vi "test-FlyWheel-Sim-Test2.vi"() -> (3 "All Passed":bool)   [LabVIEW 2019]
uses:
  <vilib>/Analysis/Matrix/Datatypes/RealMatrix.ctl
  <vilib>/Analysis/Matrix/NI_Matrix.lvlib
  <vilib>/Rock Robotics/WPI/ThirdParty/JAS_Junk/TrajLib/Trajectory_Library.lvlib
  <vilib>/Rock Robotics/WPI/ThirdParty/JAS_Junk/TrajLib/DCMotor_GetCIM.vi
panel:
  out "Speed Control Passed":bool
  out "Speed Ctrl":T1(graph)
  out "Error":bool
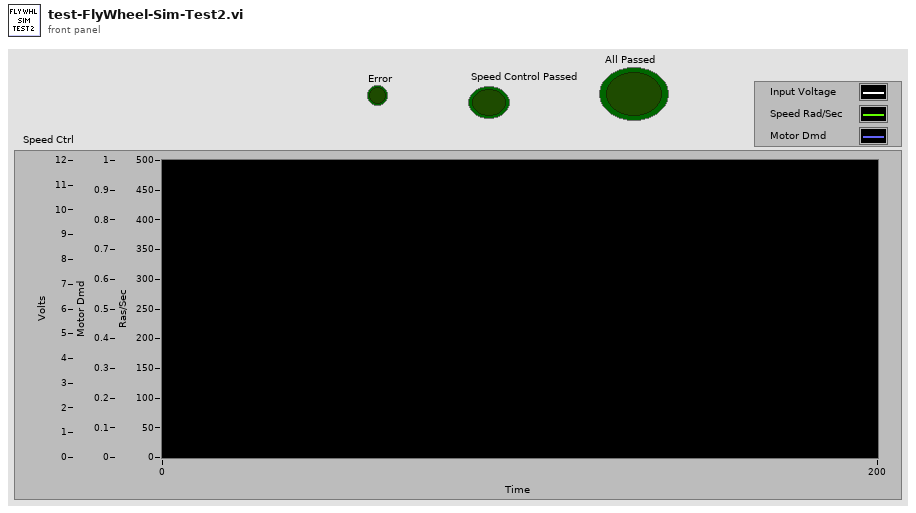
[diagram p1: front panel]
types:
  T1 = cluster{dbl, "Velocity_RadPerSec":dbl, "upper limit":dbl}
  T2 = typedef "NI_Matrix.lvlib/RealMatrix.ctl" = dbl[][]
  T3 = typedef "Trajectory_Library.lvlib/DCMOTOR.CTL" = cluster{"nominalVoltage_Volts":dbl, "StallTorque_NM":dbl, "StallCurrent_Amps":dbl, "FreeCurrent_Amps":dbl, "FreeSpeed_RadPerSec":dbl, "R_Ohms":dbl, "KvINV_RadPerSecPerVolt":dbl, "Kt_NMPerAmp":dbl, "L_H":dbl, "Jr_KgM2":dbl}
  T4 = typedef "Trajectory_Library.lvlib/FLYWHEEL_SIM.ctl" = cluster{"LinearSystemSim":T5, "GearBox":T3, "Gearing":dbl}
  T5 = typedef "Trajectory_Library.lvlib/LINEAR_SYSTEM_SIM.ctl" = cluster{"m_Plant":T6, "m_X":T2, "m_Y":T2, "m_U":T2, "MeasureStdDev":T2}
  T6 = typedef "Trajectory_Library.lvlib/LINEAR_SYSTEM.ctl" = cluster{"m_A":T2, "m_B":T2, "m_C":T2, "m_D":T2, "States":i32, "Inputs":i32, "Outputs":i32}
  T7 = typedef "Trajectory_Library.lvlib/PID_TUNING.ctl" = cluster{"Kp":dbl, "Ki":dbl, "Kd":dbl, "MaximumIntegral":dbl, "MinimumIntegral":dbl, "IntegralZone":dbl}
  T8 = typedef "Trajectory_Library.lvlib/PID_INPUT_LIMITS.ctl" = cluster{"MaxInput":dbl, "MinInput":dbl, "Continuous":bool}
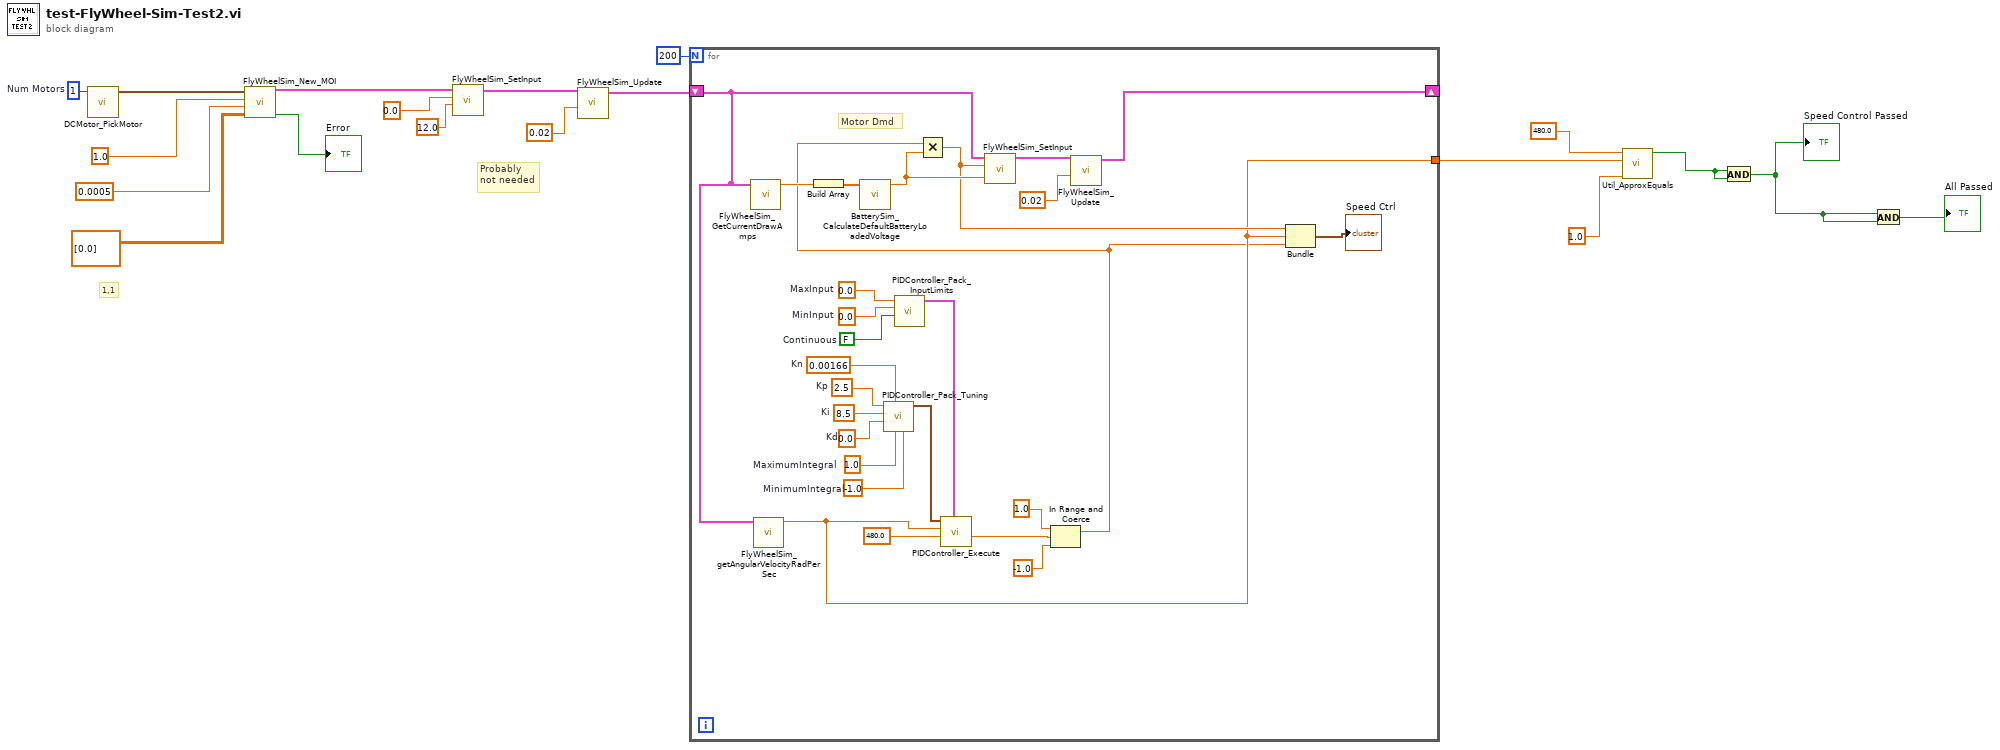
[diagram p0: block diagram]
diagram:
  w19 = 1  # Num Motors
  # "Probably \nnot needed"
  # "1,1"
  n1 = call-poly <vilib>:"DCMotor_PickMotor.vi"("Num Motors"=w19) -> ("DCMOTOR"=w7:T3)  [unwired: 10 in]
  n2 = call <vilib>:"FlyWheelSim_New_MOI.vi"("MeasurementStdDev"=T2 [[0.0]], "jKgMetersSquared"=0.0005, "Gearing"=1.0, "GearBox"=w7) -> ("Error"=→"Error":bool, "FlyWheelSim"=w13:T4)  [unwired: 6 in]
  n3 = call <vilib>:"FlyWheelSim_SetInput.vi"("Battery_Volts"=12.0, "Volts"=0.0, "FlyWheelSim"=w13) -> ("out FlyWheelSim"=w9:T4)  [unwired: 8 in]
  n4 = call <vilib>:"FlyWheelSim_Update.vi"("dT_Seconds"=0.02, "FlyWheelSim"=w9) -> ("out FlyWheelSim"=w8:T4)  [unwired: 8 in, 1 out]
  n5 = for {
    N: 200 -> [_]
    shift-right: [w38] -> _
    shift-left: w8 -> [w25]
    tunnel: [w21] -> w2
    w37 = 0.00166  # Kn
    w36 = 0.0  # MaxInput
    w35 = 0.0  # MinInput
    w34 = FALSE  # Continuous
    w33 = 2.5  # Kp
    w32 = 8.5  # Ki
    w31 = 0.0  # Kd
    w30 = 1.0  # MaximumIntegral
    w29 = -1.0  # MinimumIntegral
    # "Motor Dmd"
    n6 = call <vilib>:"FlyWheelSim_GetCurrentDrawAmps.vi"("FlyWheelSim"=w25) -> ("Current_Amps"=w44:dbl)  [unwired: 10 in]
    n7 = call <vilib>:"FlyWheelSim_getAngularVelocityRadPerSec.vi"("FlyWheelSim"=w25) -> ("Velocity_RadPerSec"=w21:dbl)  [unwired: 10 in]
    n8 = Build Array(w44) -> (w45:dbl[])
    n9 = call <vilib>:"BatterySim_CalculateDefaultBatteryLoadedVoltage.vi"("Currents"=w45) -> ("Voltage"=w43:dbl)  [unwired: 10 in]
    n10 = call <vilib>:"PIDController_Pack_Tuning.vi"("MinimumIntegral"=w29, "MaximumIntegral"=w30, "Kn"=w37, "Kd"=w31, "Ki"=w32, "Kp"=w33) -> ("PID Tuning"=w28:T7)  [unwired: 5 in]
    n11 = call <vilib>:"PIDController_Pack_InputLimits.vi"("Continuous"=w34, "MinInput"=w35, "MaxInput"=w36) -> ("PID Input Limits"=w27:T8)  [unwired: 8 in]
    n12 = call <vilib>:"PIDController_Execute.vi"("PID Input Limits"=w27, "SP-SetPoint"=480.0, "PV-Measurement"=w21, "PID Tuning"=w28) -> ("CO-ControlOutput"=w22:dbl)  [unwired: 5 in, 2 out]
    n13 = In Range and Coerce(upper limit=1.0, x=w22, lower limit=-1.0) -> (coerced(x)=w20:dbl)  [unwired: 1 out]
    n14 = Multiply(x=w20, y=w43) -> (x*y=w39:dbl)
    n15 = call <vilib>:"FlyWheelSim_SetInput.vi"("Battery_Volts"=w43, "Volts"=w39, "FlyWheelSim"=w25) -> ("out FlyWheelSim"=w42:T4)  [unwired: 8 in]
    n16 = call <vilib>:"FlyWheelSim_Update.vi"("dT_Seconds"=0.02, "FlyWheelSim"=w42) -> ("out FlyWheelSim"=w38:T4)  [unwired: 8 in, 1 out]
    n17 = Bundle(w39, "Velocity_RadPerSec"=w21, "upper limit"=w20) -> (→"Speed Ctrl":T1)  [unwired: 1 in]
  }
  n18 = call <vilib>:"Util_ApproxEquals.vi"("Tolerance"=1.0, "Value 2"=w2, "Value 1"=480.0 ("y")) -> ("ApproxEquals"=w1:bool)  [unwired: 8 in]
  n19 = And(x=w1, y=w1) -> (x .and. y?=w3:bool)
  "Speed Control Passed" <- w3
  n20 = And(x=w3, y=w3) -> (x .and. y?=→"All Passed":bool)
